vi "appendXMLROI.vi"(0 "DOM document in":refnum<k20>, 1 "Parent Camera Node":refnum<k20>, 2 "error in (no error)":errorcluster, 3 "ROI":i32[](array[numeric])) -> (10 "error out":errorcluster)   [LabVIEW 2013]
uses:
  <resource>/objmgr/DOMUserDefRef.rc
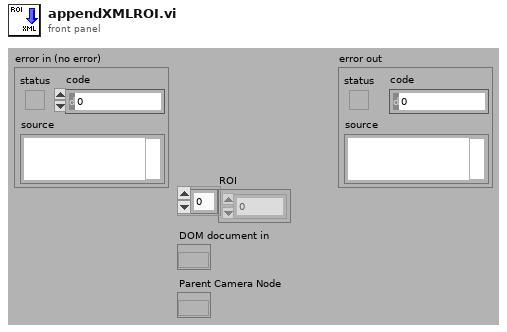
[diagram p1: front panel]
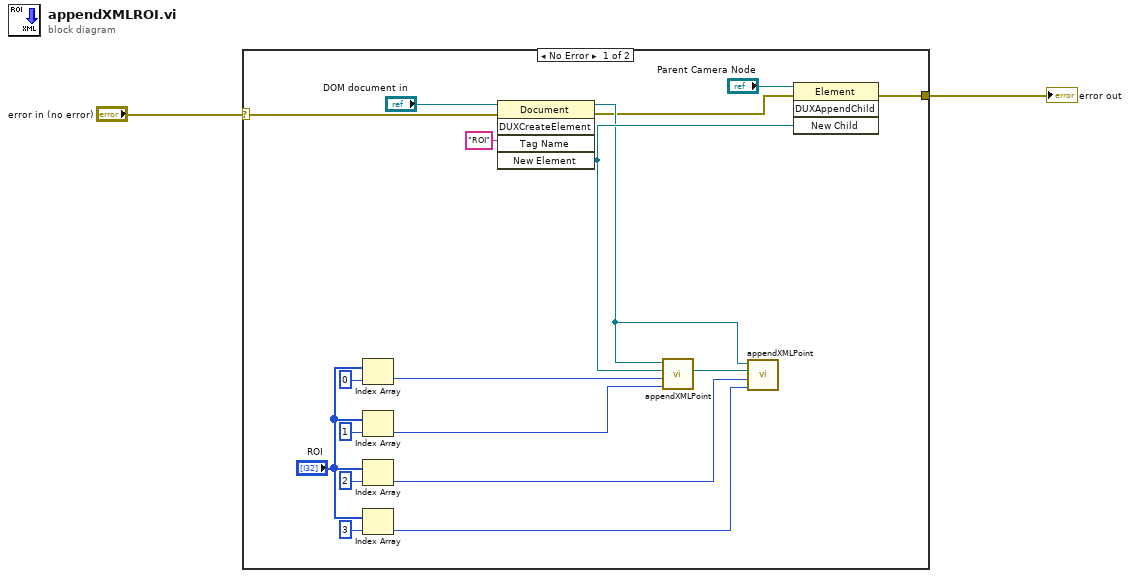
[diagram p0: block diagram]
diagram:
  n1 = case shown="No Error" "error in (no error)" {
    selector: "error in (no error)" -> [w3 w21]
    tunnel: [w4 w21] -> w2
    frame No Error {
      n2 = Index Array(array="ROI", index=0) -> (element=w20:i32)
      n3 = Index Array(array="ROI", index=1) -> (element=w19:i32)
      n4 = Index Array(array="ROI", index=2) -> (element=w17:i32)
      n5 = Index Array(array="ROI", index=3) -> (element=w16:i32)
      n6 = invoke class="Document" method="DUXCreateElement"(reference="DOM document in", error in=w3, "Tag Name"="ROI") -> (reference out=w6:refnum<k20>, error out=w5:errorcluster, "New Element"=w7:refnum<k20>)  [unwired: 2 in, 2 out]
      n7 = call "appendXMLPoint.vi"("y"=w19, "x"=w20, "Parent Node"=w7, "DOM document in"=w6) -> ("Parent Node Out"=w11:refnum<k20>)  [unwired: 5 in, 1 out]
      n8 = call "appendXMLPoint.vi"("y"=w16, "x"=w17, "Parent Node"=w11, "DOM document in"=w6) -> ()  [unwired: 5 in, 2 out]
      n9 = invoke class="Element" method="DUXAppendChild"(reference="Parent Camera Node", error in=w5, "New Child"=w7) -> (error out=w4:errorcluster)  [unwired: 1 in, 3 out]
    }
    frame Error {
    }
  }
  "error out" <- w2
